vi "liblinear_predict.vi"(8 "error in (no error)":errorcluster, 10 "x":T1[](array[typedef]), 11 "liblinear_model":T2={"liblinear_parameter"={"solver_type"=0, "eps"=0.01, "C"=1.0, "weight_label"=[], "weight"=[], "p"=0.1}, "nr_class"=0, "nr_feature"=0, "w"=[], "label"=[], "bias"=0.0} {"liblinear_parameter"."solver_type" items=["L2R_LR"=0, "L2R_L2LOSS_SVC_DUAL"=1, "L2R_L2LOSS_SVC"=2, "L2R_L1LOSS_SVC_DUAL"=3, "MCSVM_CS"=4, "L1R_L2LOSS_SVC"=5, "L1R_LR"=6, "L2R_LR_DUAL"=7, "L2R_L2LOSS_SVR"=11, "L2R_L2LOSS_SVR_DUAL"=12, "L2R_L1LOSS_SVR_DUAL"=13]}) -> (0 "error out":errorcluster, 3 "predicted label":dbl)   [LabVIEW 2015]
uses:
  Controls/liblinear_model.ctl
  Controls/liblinear_parameter.ctl
  Controls/liblinear_solver.ctl
  LibSVM Sparse/Wrapper API/Controls/svm_node.ctl
  bin/x64/LabVIEW-liblinear.dll
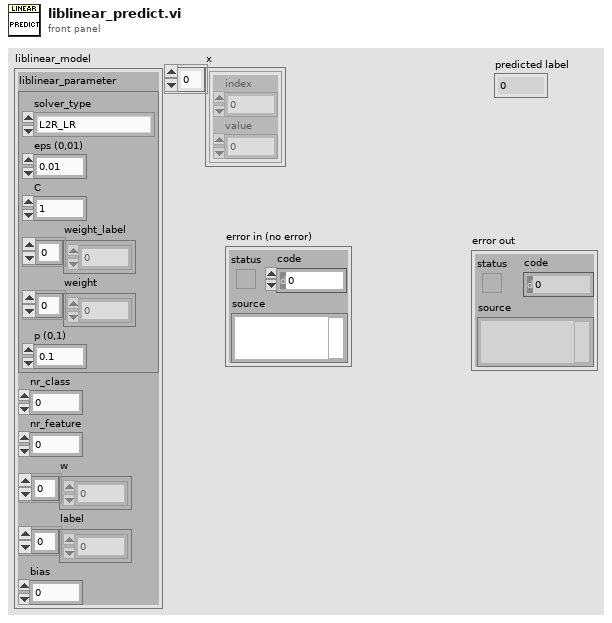
[diagram p1: front panel]
types:
  T1 = typedef "svm_node.ctl" = cluster{"index":i32, "value":dbl}
  T2 = typedef "liblinear_model.ctl" = cluster{"liblinear_parameter":T3, "nr_class":i32, "nr_feature":i32, "w":dbl[], "label":i32[], "bias":dbl}
  T3 = typedef "liblinear_parameter.ctl" = cluster{"solver_type":T4, "eps":dbl, "C":dbl, "weight_label":i32[], "weight":dbl[], "p":dbl}
  T4 = typedef "liblinear_solver.ctl" = u32
  T5 = typedef "svm_node_padded.ctl" = cluster{"index":i32, "padding":i32, "value":dbl}
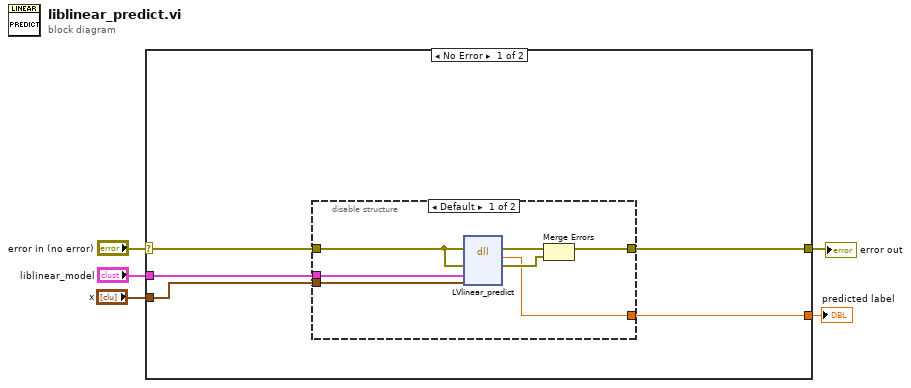
[diagram p0: block diagram]
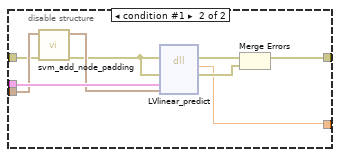
[diagram p2: hidden frame]
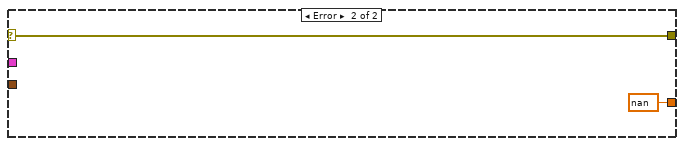
[diagram p3: hidden frame]
diagram:
  n1 = case shown="No Error" "error in (no error)" {
    selector: "error in (no error)" -> [w10 w28]
    tunnel: [w9 w28] -> w5
    tunnel: "liblinear_model" -> [w8 _]
    tunnel: "x" -> [w7 _]
    tunnel: [w6 nan ("predicted label")] -> w1
    frame No Error {
      n2 = disable-structure shown="Default" {
        disable-tunnel: w10 -> [w17 w18]
        disable-tunnel: [w15 w25] -> w9
        disable-tunnel: w8 -> [w13 w23]
        disable-tunnel: w7 -> [w12 w21]
        disable-tunnel: [w11 w22] -> w6
        frame condition #0 (active) {
          n3 = dll-call lib="C:/dev/LabVIEW-libsvm/LabVIEW/bin/x64/LabVIEW-liblinear.*" fn="LVlinear_predict"(error in=w17, "lvErr"=w17, "model_in"=w13, "x_in"=w12) -> (error out=w16:errorcluster, "predicted label"=w11:dbl, "lvErr"=w14:errorcluster)  [unwired: 4 in, 1 out]
          n4 = Merge Errors(w16, w14) -> (w15:errorcluster)
        }
        frame condition #1 {
          n5 = call "svm_add_node_padding.vi"("error in (no error)"=w18, "Nodes"=w21) -> ("error out"=w19:errorcluster, "Padded nodes"=w20:T5[])  [unwired: 8 in]
          n6 = dll-call lib="C:/dev/LabVIEW-libsvm/LabVIEW/bin/x64/LabVIEW-liblinear.*" fn="LVlinear_predict"(error in=w19, "lvErr"=w19, "model_in"=w23, "x_in"=w20) -> (error out=w26:errorcluster, "predicted label"=w22:dbl, "lvErr"=w24:errorcluster)  [unwired: 4 in, 1 out]
          n7 = Merge Errors(w26, w24) -> (w25:errorcluster)
        }
      }
    }
    frame Error {
    }
  }
  "error out" <- w5
  "predicted label" <- w1
